vi "goStraight.vi"(0 "KickToSkill in":refnum<class "KickToSkill.lvclass">, 1 "Target":dbl[](array[numeric]), 5 "Raio":dbl=123.0, 7 "Game":refnum<class "Game.lvclass">, 9 "Robot in":refnum<class "Robot.lvclass">, 11 "error in (no error)":errorcluster) -> (4 "KickToSkill out":refnum<class "KickToSkill.lvclass">, 6 "Robot out":refnum<class "Robot.lvclass">, 15 "error out":errorcluster)   [LabVIEW 2023, in "KickToSkill.lvclass"]
uses:
  KickToSkill.lvclass
  Robot_class/Robot.lvclass
  Game_class/Game.lvclass
  Game_class/Game.lvclass/Game.ctl
  Object_class/Object.lvclass/Object.ctl
  Robot_class/Robot.lvclass/Robot.ctl
  Game_class/Read BallRef.vi
  Object_class/Read position(x,y).vi
  Robot_class/Write dest_x.vi
  Robot_class/Write dest_y.vi
  Robot_class/Write dest_orientation.vi
  Ball_class/Ball.lvclass
  C:/Users/ebert/Desktop/roboime/SSL_AI/Object_class/Object.lvclass
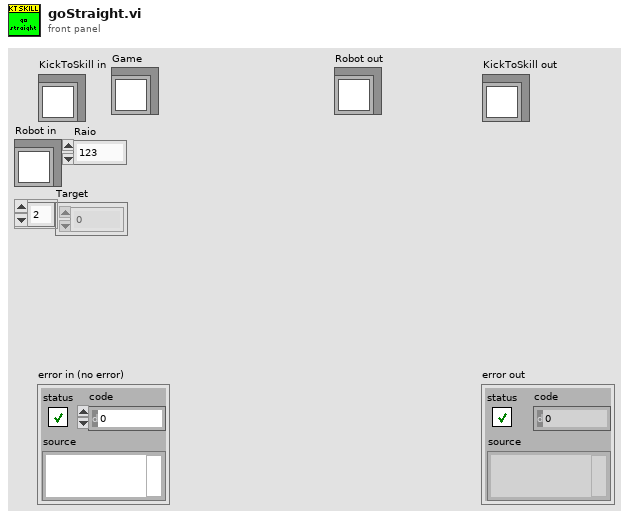
[diagram p1: front panel]
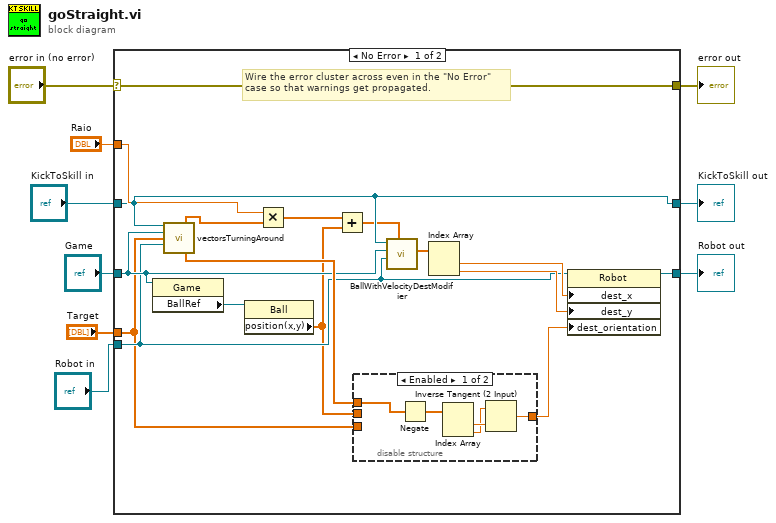
[diagram p0: block diagram]
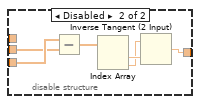
[diagram p2: hidden frame]
diagram:
  n1 = case shown="No Error" "error in (no error)" {
    selector: "error in (no error)" -> [w26 w40]
    tunnel: [w26 w40] -> w8
    tunnel: [w16 w39] -> w6
    tunnel: "KickToSkill in" -> [w16 w39]
    tunnel: "Robot in" -> [w14 w38]
    tunnel: [w25 w38] -> w4
    tunnel: "Game" -> [w15 _]
    tunnel: "Target" -> [w11 _]
    tunnel: "Raio" -> [w17 _]
    frame No Error {
      # "Wire the error cluster across even in the \"No Error\"\ncase so that warnings get propagated."
      n2 = property class="Game"(reference=w15) -> ("BallRef"=w24:refnum<class "Ball.lvclass">)  [unwired: 1 in, 2 out]
      n3 = call "vectorsTurningAround.vi"("KickToSkill in"=w16, "Game"=w15, "Target"=w11, "Robot in"=w14) -> ("Ball - Target"=w18:dbl[], "Robot - Ball"=w20:dbl[])  [unwired: 4 in, 6 out]
      n4 = property class="Ball"(reference=w24) -> ("position(x,y)"=w10:dbl[])  [unwired: 1 in, 2 out]
      n5 = Multiply(x=w17, y=w18) -> (x*y=w23:dbl[])
      n6 = Add(x=w23, y=w10) -> (x+y=w13:dbl[])
      n7 = disable-structure shown="Enabled" {
        disable-tunnel: w20 -> [w31 _]
        disable-tunnel: [w27 w33] -> w19
        disable-tunnel: w11 -> [_ w35]
        disable-tunnel: w10 -> [_ w34]
        frame Enabled {
          n8 = Negate(x=w31) -> (-x=w30:dbl[])
          n9 = Index Array(array=w30) -> (element #1=w29:dbl, element #2=w28:dbl)  [unwired: 2 in]
          n10 = Inverse Tangent (2 Input)(1:w29, 2:w28) -> (0:w27:dbl)
        }
        frame Disabled {
          n11 = Subtract(x=w35, y=w34) -> (x-y=w36:dbl[])
          n12 = Index Array(array=w36) -> (element #1=w37:dbl, element #2=w32:dbl)  [unwired: 2 in]
          n13 = Inverse Tangent (2 Input)(1:w37, 2:w32) -> (0:w33:dbl)
        }
      }
      n14 = call "BallWithVelocityDestModifier.vi"("destino original"=w13, "Robot in"=w14, "Game"=w15, "KickToSkill in"=w16) -> ("destino com velocidade"=w12:dbl[])  [unwired: 5 in, 2 out]
      n15 = Index Array(array=w12) -> (element #1=w22:dbl, element #2=w21:dbl)  [unwired: 2 in]
      n16 = property class="Robot"(reference=w14, "dest_x"=w22, "dest_y"=w21, "dest_orientation"=w19) -> (reference out=w25:refnum<class "Robot.lvclass">)  [unwired: 1 in, 1 out]
    }
    frame Error {
    }
  }
  "error out" <- w8
  "KickToSkill out" <- w6
  "Robot out" <- w4
